vi "GOOP4_Sub_Create.vi"(8 "error in (no error)":errorcluster, 9 "Str":string, 10 "i":i32, 11 "reference in":refnum<class "GOOP4_Sub.lvclass">) -> (0 "error out":errorcluster, 3 "reference out":refnum<class "GOOP4_Sub.lvclass">)   [LabVIEW 2019, in "GOOP4_Sub.lvclass"]
uses:
  GOOP4_Sub.lvclass
  C:/Users/Tiba/Desktop/1GOOP4_CreateObjects_Open_GDS/GOOP4_Base_class/GOOP4_Base.lvclass
  GOOP4_Sub.lvclass/GOOP4_Sub.ctl
  GOOP4_Sub_AAAa_interface/GOOP4_Sub_AAAa.lvclass
  C:/Users/Tiba/Desktop/1GOOP4_CreateObjects_Open_GDS/AAAa_Interface/AAAa.lvclass
  GOOP4_Base_class/GOOP4_Base.lvclass
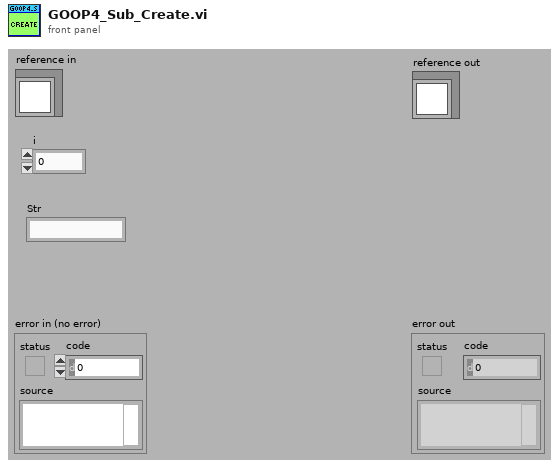
[diagram p1: front panel]
types:
  T1 = typedef "GOOP4_Sub.lvclass/ObjectAttributes.ctl" = cluster{"Str":string, "Boolean":bool}
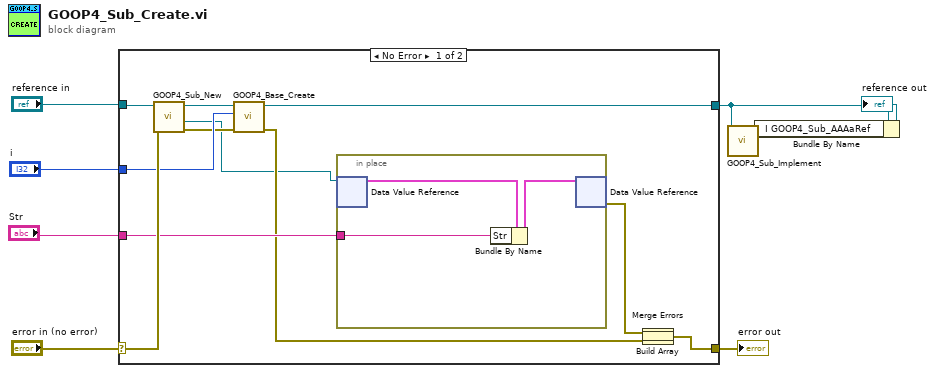
[diagram p0: block diagram]
diagram:
  n1 = case shown="No Error" "error in (no error)" {
    selector: "error in (no error)" -> [w19 w25]
    tunnel: [w17 w25] -> w7
    tunnel: "reference in" -> [w20 w24]
    tunnel: [w12 w24] -> w2
    tunnel: "i" -> [w16 _]
    tunnel: "Str" -> [w15 _]
    frame No Error {
      n2 = call "GOOP4_Sub_New.vi"("error in (no error)"=w19, "reference in"=w20) -> ("error out"=w11:errorcluster, "DVRRefOut"=w9:refnum<data-value>, "reference out"=w13:refnum<class "GOOP4_Sub.lvclass">)  [unwired: 6 in, 1 out]
      n3 = call "GOOP4_Base_Create.vi"("error in (no error)"=w11, "i"=w16, "reference in"=w13) -> ("error out"=w10:errorcluster, "reference out"=w12:refnum<class "GOOP4_Sub.lvclass">)  [unwired: 7 in]
      n4 = in-place {
        in-place-border: w15 -> [w21]
        n5 = in-place-dvr #1(w9) -> (w22:T1)  [unwired: 1 out]
        n6 = Bundle By Name(cluster=w22, "Str"=w21) -> (w23:T1)
        n7 = in-place-dvr #1(w23) -> (w18:errorcluster)  [unwired: 1 out]
      }
      n8 = Build Array(w18, w10) -> (w14:errorcluster[])
      n9 = Merge Errors(w14) -> (w17:errorcluster)
    }
    frame Error {
    }
  }
  "error out" <- w7
  n10 = call "GOOP4_Sub_Implement.vi"("ClassThatImplements"=w2) -> ("InterfaceHelpClass"=w1:refnum<class "GOOP4_Sub_AAAa.lvclass">)  [unwired: 10 in]
  n11 = Bundle By Name(cluster=w2, "I GOOP4_Sub_AAAaRef"=w1) -> (→"reference out":refnum<class "GOOP4_Sub.lvclass">)
